vi "test_i32 (Missing).vi"(8 "error in (no error)":errorcluster, 11 "TestCase in":refnum<class "Test Read File.lvclass">) -> (0 "error out":errorcluster, 3 "TestCase out":refnum<class "Test Read File.lvclass">)   [LabVIEW 2019, in "Test Read File.lvclass"]
uses:
  Test Read File.lvclass
  C:/Program Files/National Instruments/LabVIEW 2024/vi.lib/Astemes/LUnit/Test Case.lvclass
  Test Read File.lvclass/Test Read File.ctl
  <vilib>/Astemes/LUnit/Test Case.lvclass/Test Case.ctl
  f5d29829-c36f-4d55-a638-6f2da4fc6c93.vi
  <vilib>/Astemes/LUnit/Core/LUnit Test Case/Private/Append Pass Result.vi
  <vilib>/Astemes/LUnit/Core/LUnit Test Case/Private/Append Fail Result.vi
  f5d29829-c36f-4d55-a638-6f2da4fc6c93.vi/9c5d11cd-9439-4240-a1ee-d9baace9c924.vi
  <vilib>/Astemes/LUnit/Core/LUnit Test Case/Private/Run In UI.vi
  <vilib>/Utility/error.llb/Clear Errors.vi
  Read/Read Section - I32.vi
  TSC File IO.lvlib
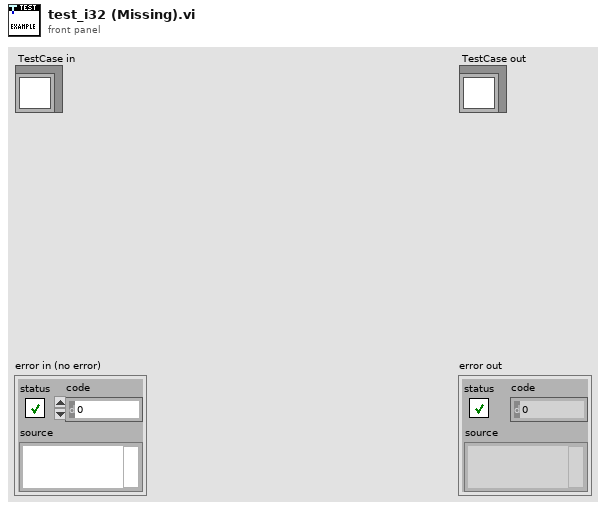
[diagram p1: front panel]
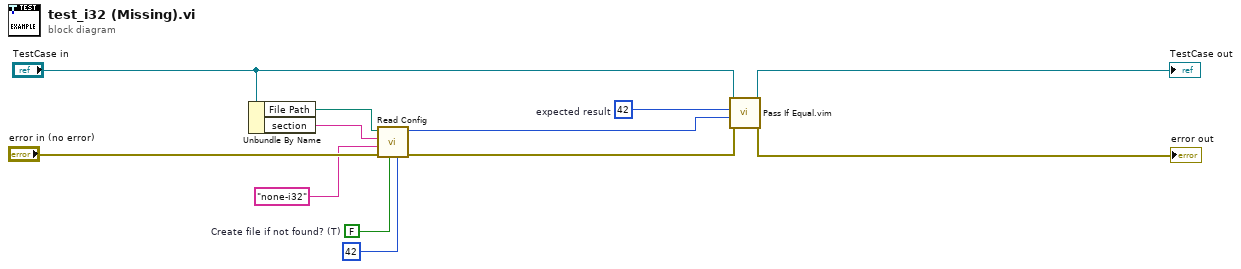
[diagram p0: block diagram]
diagram:
  w2 = FALSE  # Create file if not found? (T)
  w8 = 42  # expected result
  n1 = Unbundle By Name("TestCase in") -> ("File Path"=w6:path, "section"=w5:string)
  n2 = call-poly "Read Config.vi"("Default"=42, "Create file if not found? (T)"=w2, "error in (no error)"="error in (no error)", "key"="none-i32", "section"=w5, "Path"=w6) -> ("error out"=w7:errorcluster, "value"=w4:i32)  [unwired: 4 in]
  n3 = call "Pass If Equal.vim"("error in (no error)"=w7, "Actual"=w4, "Expected"=w8, "LUnit Test Case In"="TestCase in") -> ("error out"=→"error out":errorcluster, "LUnit Test Case Out"=→"TestCase out":refnum<class "Test Read File.lvclass">)  [unwired: 6 in]
